vi "Get Available List.vi"(7 "list property name":string, 8 "error in (no error)":errorcluster, 9 "GUID.Main Disabled":string, 10 "GUID.Main Enabled":string, 11 "Item Ref in":T1 format="%.0x") -> (0 "error out":errorcluster, 2 "available items":string[](array[string]), 3 "Item Ref out":T1 format="%.0x")   [LabVIEW 2020]
uses:
  <vilib>/NI VeriStand/Custom Device API/Custom Device Item Ref.ctl
  <vilib>/NI VeriStand/Custom Device Tools/Custom Device Utility Library/Search Direction.ctl
  <vilib>/NI VeriStand/Custom Device Tools/Custom Device Utility Library/NI VeriStand - Search for Item by GUID.vi
  <vilib>/NI VeriStand/Custom Device API/Get Item Property (String Array).vi
  <vilib>/NI VeriStand/Custom Device Tools/Custom Device Utility Library/Custom Device Utility Library.lvlib
  <vilib>/NI VeriStand/Custom Device API/Custom Device API.lvlib
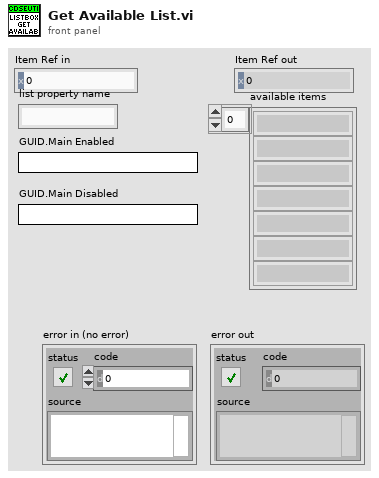
[diagram p1: front panel]
types:
  T1 = typedef "Custom Device API.lvlib/Custom Device Item Ref.ctl" = u64
  T2 = typedef "Custom Device Utility Library.lvlib/Search Direction.ctl" = enum16{"Down", "Up"}
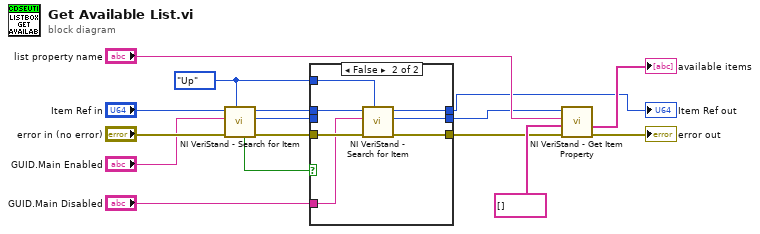
[diagram p0: block diagram]
diagram:
  w6 = Search_Direction."Up" ("Direction (Down)")
  n1 = call-poly <vilib>:"NI VeriStand - Search for Item.vi"("Direction (Down)"=w6, "error in"="error in (no error)", "Item GUID"="GUID.Main Enabled", "Section Ref in"="Item Ref in") -> ("error out"=w9:errorcluster, "Item Ref"=w7:T1, "Section Ref out"=w8:T1, "Found"=w10:bool)  [unwired: 4 in]
  n2 = case shown="False" w10 {
    tunnel: w9 -> [w19 w26]
    tunnel: w8 -> [w17 w25]
    tunnel: w7 -> [w18 _]
    tunnel: "GUID.Main Disabled" -> [_ w24]
    tunnel: w6 -> [_ w23]
    tunnel: [w18 w22] -> w5
    tunnel: [w17 w21] -> w4
    tunnel: [w19 w20] -> w3
    frame True {
    }
    frame False {
      n3 = call-poly <vilib>:"NI VeriStand - Search for Item.vi"("Direction (Down)"=w23, "error in"=w26, "Item GUID"=w24, "Section Ref in"=w25) -> ("error out"=w20:errorcluster, "Item Ref"=w22:T1, "Section Ref out"=w21:T1)  [unwired: 4 in, 1 out]
    }
  }
  "Item Ref out" <- w4
  n4 = call-poly <vilib>:"NI VeriStand - Get Item Property.vi"("error in (no error)"=w3, "Default Value"=string[] [], "Property Name"="list property name", "Item Ref in"=w5) -> ("error out"=→"error out":errorcluster, "Value"=→"available items":string[])  [unwired: 4 in, 2 out]
